vi "Save_Positions.vi"(1 "Cordinates":T2 {"Schritte B" format="%#.4g"; "Schritte A" format="%#.4g"; "Schritte C" format="%#.4g"; "Schritte U" format="%#.4g"; "Schritte Z" format="%#.4g"; "Schritte Y" format="%#.4g"; "Schritte X" format="%#.4g"}, 2 "Position":T1(ring), 3 "Boolean":bool) -> (0 "Array":sgl[](array[numeric]))   [LabVIEW 2013]
panel:
  in  "Array 2":sgl[](array[numeric])
  out "P10":dbl[](array[numeric])
  out "P9":dbl[](array[numeric])
  out "P8":dbl[](array[numeric])
  out "P6":dbl[](array[numeric])
  out "P5":dbl[](array[numeric])
  out "P4":dbl[](array[numeric])
  out "P7":dbl[](array[numeric])
  out "P3":dbl[](array[numeric])
  out "P2":dbl[](array[numeric])
  out "P1":dbl[](array[numeric])
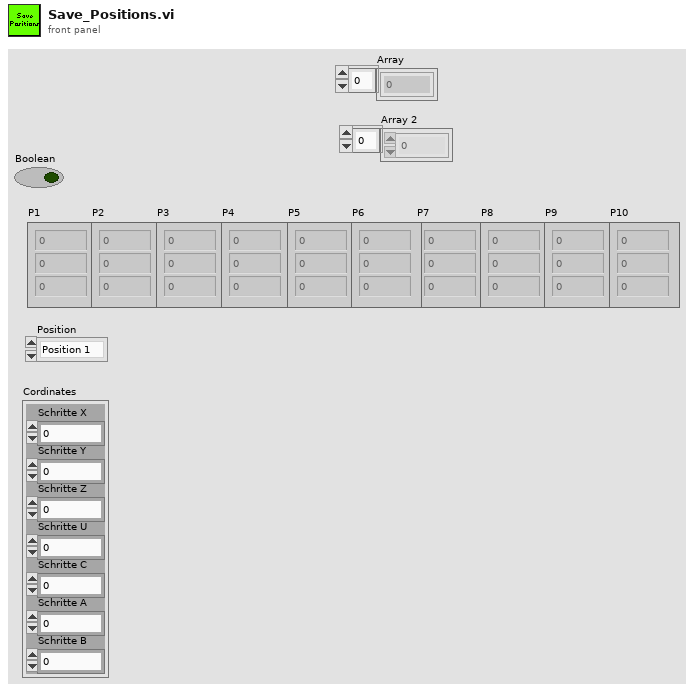
[diagram p1: front panel]
types:
  T1 = enum16{"Position 1", "Position 2", "Position 3", "Position 4", "Position 5", "Position 6", "Position 7", "Position 8", "Position 9", "Position 10"}
  T2 = cluster{"Schritte X":sgl, "Schritte Y":sgl, "Schritte Z":sgl, "Schritte U":sgl, "Schritte C":sgl, "Schritte A":sgl, "Schritte B":sgl}
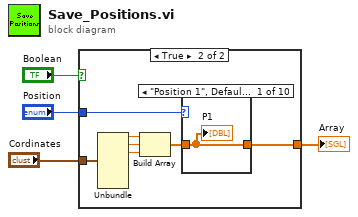
[diagram p0: block diagram]
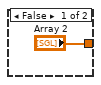
[diagram p2: hidden frame]
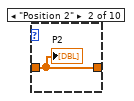
[diagram p3: hidden frame]
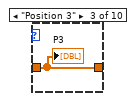
[diagram p4: hidden frame]
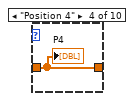
[diagram p5: hidden frame]
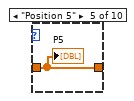
[diagram p6: hidden frame]
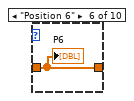
[diagram p7: hidden frame]
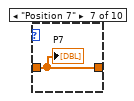
[diagram p8: hidden frame]
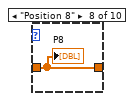
[diagram p9: hidden frame]
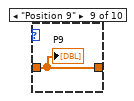
[diagram p10: hidden frame]
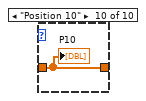
[diagram p11: hidden frame]
diagram:
  n1 = case shown="True" "Boolean" {
    tunnel: "Position" -> [_ w8]
    tunnel: "Cordinates" -> [_ w7]
    tunnel: ["Array 2" w6] -> w1
    frame False {
    }
    frame True {
      n2 = Unbundle(w7) -> ("Schritte X"=w12:sgl, "Schritte Y"=w11:sgl, "Schritte Z"=w10:sgl)  [unwired: 4 out]
      n3 = Build Array(w12, w11, w10) -> (w9:sgl[])
      n4 = case shown="\"Position 1\", Default" w8 {
        tunnel: w9 -> [w13 w14 w15 w16 w17 w18 w19 w20 w21 w22]
        tunnel: [w13 w14 w15 w16 w17 w18 w19 w20 w21 w22] -> w6
        frame "Position 1", Default {
          "P1" <- w13
        }
        frame "Position 2" {
          "P2" <- w14
        }
        frame "Position 3" {
          "P3" <- w15
        }
        frame "Position 4" {
          "P4" <- w16
        }
        frame "Position 5" {
          "P5" <- w17
        }
        frame "Position 6" {
          "P6" <- w18
        }
        frame "Position 7" {
          "P7" <- w19
        }
        frame "Position 8" {
          "P8" <- w20
        }
        frame "Position 9" {
          "P9" <- w21
        }
        frame "Position 10" {
          "P10" <- w22
        }
      }
    }
  }
  "Array" <- w1
